vi "subvicomp.vi"() -> ()   [LabVIEW 2021]
panel:
  in  "1.4":dbl
  in  "1.3":dbl
  in  "1.2":dbl
  out "2":dbl
  in  "1":dbl
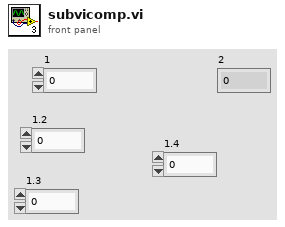
[diagram p1: front panel]
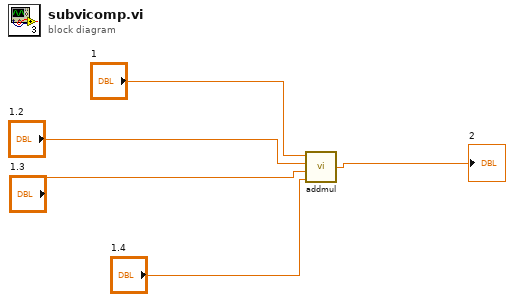
[diagram p0: block diagram]
diagram:
  n1 = call "addmul.vi"("Numeric 4"="1.4", "Numeric 3"="1.3", "Numeric 2"="1.2", "Numeric"="1") -> ("Numeric 5"=→"2":dbl)
